vi "Order Spectrum (Analog Tach).vi"(5 "window type":T2(ring)=enum."Hanning", 7 "dB On (T)":bool=TRUE, 8 "pulse/revolution (1)":i32=1, 9 "analog tach signal":waveform(dbl)={"t0"=timestamp(0 s since 1904-01-01), "dt"=0.0, "Y"=[]}, 11 "scaled signal [EU]":waveform(dbl)={"t0"=timestamp(0 s since 1904-01-01), "dt"=0.0, "Y"=[]}) -> (0 "average speed [rpm]":dbl format="%.2f", 2 "unit label":string, 3 "order spectrum":T1 {"order 0" format="%.2p"; "delta order" format="%.2p"; "magnitude" format="%.2f"})   [LabVIEW 2017]
doc: "Computes the order spectrum (power vs. orders) for <B>scaled signal </B>and <B>analog tach signal</B>."
uses:
  <vilib>/Analysis/baseanly.llb/Mean (DBL).vi
  <vilib>/addons/Sound and Vibration/Order Analysis/Backward Compatibility/OAT Sampled Power Spectrum (Single Channel).vi
  <vilib>/addons/Sound and Vibration/Order Analysis/Backward Compatibility/OAT Resample Waveform (Single Channel).vi
  <vilib>/addons/Sound and Vibration/Order Analysis/Tach Process/SoundVib_TachProcess.lvlib
  <vilib>/Analysis/NI_AALBase.lvlib
panel:
  # "Order Spectrum (Analog Tach)"
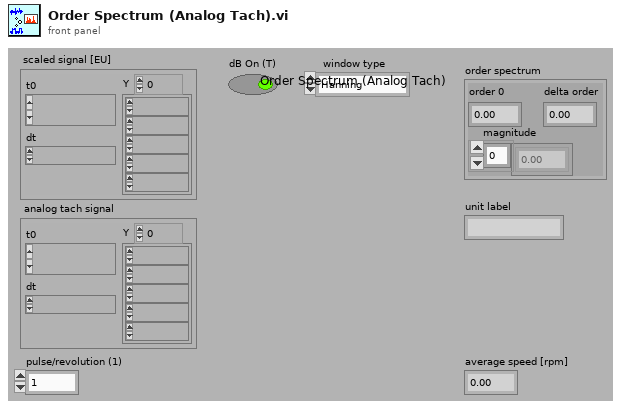
[diagram p1: front panel]
types:
  T1 = cluster{"order 0":dbl, "delta order":dbl, "magnitude":dbl[]}
  T2 = enum16{"None ", "Hanning", "Hamming", "Blackman-Harris", "Exact Blackman", "Blackman", "Flat Top", "4 Term B-Harris ", "7 Term B-Harris", "Low Sidelobe"}
  T3 = typedef "SoundVib_TachProcess.lvlib/speed profile.ctl" = cluster{"time [s]":dbl[], "speed [RPM]":dbl[]}
  T4 = cluster{"window type":enum16{"None ", "Hanning", "Hamming", "Blackman-Harris", "Exact Blackman", "Blackman", "Flat Top", "4 Term B-Harris ", "7 Term B-Harris", "Low Sidelobe"}, i32}
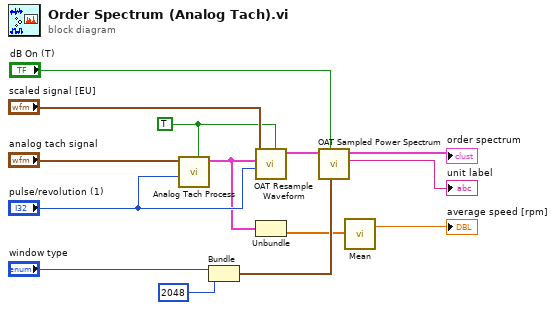
[diagram p0: block diagram]
diagram:
  w9 = TRUE ("reset? (TRUE)")
  n1 = call <vilib>:"Analog Tach Process.vi"("reset? (True)"=w9, "pulse/revolution (1)"="pulse/revolution (1)", "analog tach signal"="analog tach signal") -> ("speed profile"=w6:T3)  [unwired: 6 in, 2 out]
  n2 = Bundle("window type"="window type", 2048) -> (w8:T4)  [unwired: 1 in]
  n3 = call-poly <vilib>:"OAT Resample Waveform.vi"("reset? (True)"=w9, "pulse/revolution (1)"="pulse/revolution (1)", "speed profile"=w6, "scaled signal [EU]"="scaled signal [EU]") -> ("resampled signal"=w10:cluster{"r0":dbl, "dr":dbl, "Y":dbl[]})  [unwired: 4 in, 3 out]
  n4 = Unbundle(w6) -> ("speed [RPM]"=w5:dbl[])  [unwired: 1 out]
  n5 = call-poly <vilib>:"OAT Sampled Power Spectrum.vi"("window info"=w8, "dB On (T)"="dB On (T)", "resampled signal"=w10) -> ("unit label"=→"unit label":string, "order spectrum"=→"order spectrum":T1)  [unwired: 6 in, 1 out]
  n6 = call-poly <vilib>:"Mean.vi"("X"=w5) -> ("mean"=→"average speed [rpm]":dbl)  [unwired: 1 out]
